vi "Get Block Size.vi"(11 "Hash Function in":refnum<class "NI_SHA-256.lvclass">) -> (2 "block size (bytes)":i32, 3 "Hash Function out":refnum<class "NI_SHA-256.lvclass">)   [LabVIEW 2013, in "NI_SHA-256(2013).lvlib" / "NI_SHA-256.lvclass"]
doc: "Returns the input block size of the hash function in bytes."
uses:
  NI_SHA-256.lvclass
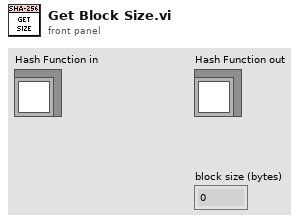
[diagram p1: front panel]
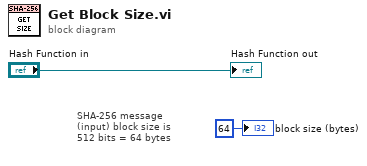
[diagram p0: block diagram]
diagram:
  # "SHA-256 message (input) block size is 512 bits = 64 bytes"
  "Hash Function out" <- "Hash Function in"
  "block size (bytes)" <- 64 ("block size (bytes)")
